vi "Unzip folder.vi"(1 "Zipped folder to unzip":path) -> (0 "Error Out":errorcluster)   [LabVIEW 2015]
uses:
  <vilib>/zip/NI_Unzip.lvlib
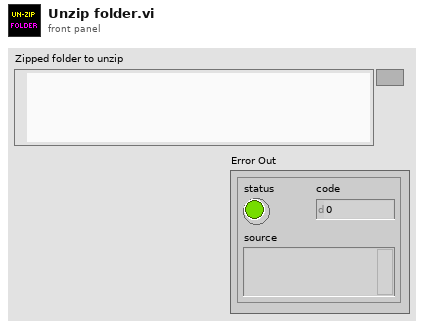
[diagram p1: front panel]
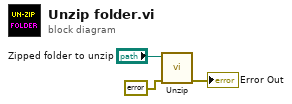
[diagram p0: block diagram]
diagram:
  n1 = call <vilib>:"Unzip.vi"("error in (no error)"=errorcluster {"status"=FALSE, "code"=0, "source"=""}, "Zip file"="Zipped folder to unzip") -> ("error out"=→"Error Out":errorcluster)  [unwired: 7 in, 2 out]
